vi "Labview_project.vi"() -> ()   [LabVIEW 2015]
panel:
  in  "Users":enum16{"1", "2", "3", "4"}(ring)
  out "Recived 4":bool
  out "Recived 3":bool
  out "Recived 1":bool
  out "Recived 2":bool
  out "Uncripted 4":bool
  out "Uncripted 3":bool
  out "Uncripted 2":bool
  out "Uncripted 1":bool
  out "User 4":dbl
  out "User 3":dbl
  out "User 2":dbl
  out "User 1":dbl
  in  "Hacked>Normal":bool
  in  "Data":dbl
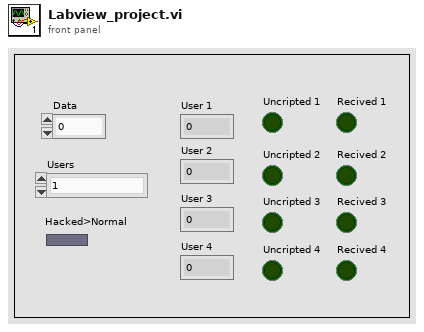
[diagram p1: front panel]
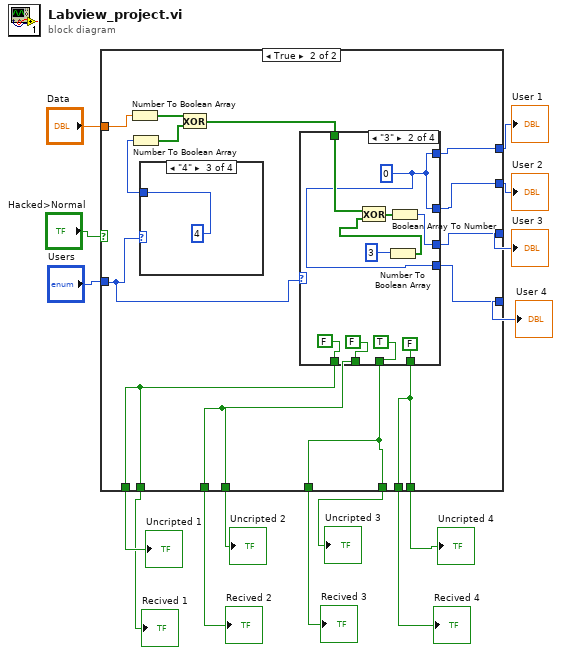
[diagram p0: block diagram]
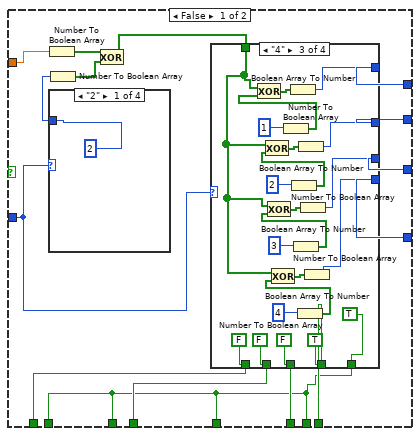
[diagram p2: hidden frame]
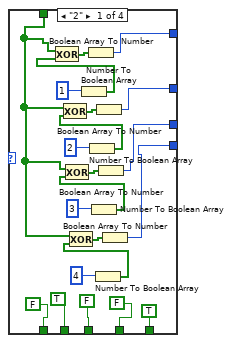
[diagram p3: hidden frame]
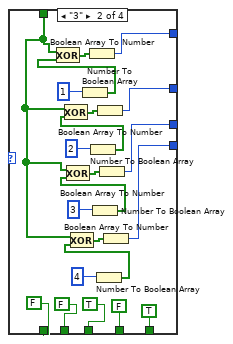
[diagram p4: hidden frame]
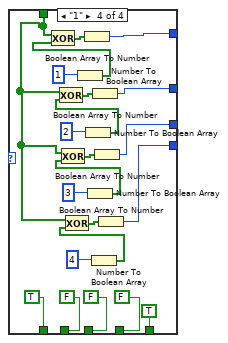
[diagram p5: hidden frame]
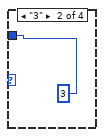
[diagram p6: hidden frame]
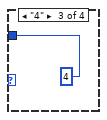
[diagram p7: hidden frame]
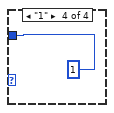
[diagram p8: hidden frame]
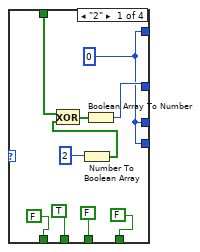
[diagram p9: hidden frame]
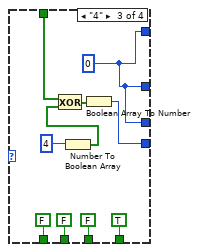
[diagram p10: hidden frame]
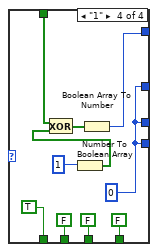
[diagram p11: hidden frame]
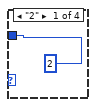
[diagram p12: hidden frame]
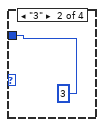
[diagram p13: hidden frame]
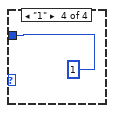
[diagram p14: hidden frame]
diagram:
  n1 = case shown="True" "Hacked>Normal" {
    tunnel: "Users" -> [w25 w132]
    tunnel: "Data" -> [w28 w134]
    tunnel: [w24 w130] -> w2
    tunnel: [w21 w129] -> w3
    tunnel: [w20 w128] -> w4
    tunnel: [w19 w127] -> w5
    tunnel: [w18 w126] -> w13
    tunnel: [w17 w125] -> w12
    tunnel: [w22 w124] -> w11
    tunnel: [w23 w123] -> w10
    tunnel: [w16 w126] -> w9
    tunnel: [w16 w125] -> w8
    tunnel: [w16 w124] -> w7
    tunnel: [w16 w123] -> w6
    frame False {
      n2 = Number To Boolean Array(number=w28) -> (Boolean array=w30:bool[])
      n3 = case shown="\"2\"" w25 {
        tunnel: [2 3 4 1] -> w27
        frame "2" {
        }
        frame "3" {
        }
        frame "4" {
        }
        frame "1" {
        }
      }
      n4 = Number To Boolean Array(number=w27) -> (Boolean array=w29:bool[])
      n5 = Exclusive Or(1:w29, 2:w30) -> (0:w26:bool[])
      n6 = case shown="\"4\"" w25 {
        tunnel: w26 -> [w36 w59 w80 w100]
        tunnel: [w32 w55 w76 w98] -> w24
        tunnel: [w33 w56 w77 w101] -> w21
        tunnel: [w34 w57 w78 w107] -> w20
        tunnel: [w35 w58 w79 w115] -> w19
        tunnel: [FALSE FALSE FALSE TRUE] -> w18
        tunnel: [TRUE FALSE FALSE FALSE] -> w17
        tunnel: [FALSE TRUE FALSE FALSE] -> w22
        tunnel: [FALSE FALSE TRUE FALSE] -> w23
        tunnel: [TRUE TRUE TRUE TRUE] -> w16
        frame "2" {
          n7 = Number To Boolean Array(number=1) -> (Boolean array=w47:bool[])
          n8 = Exclusive Or(1:w47, 2:w36) -> (0:w46:bool[])
          n9 = Boolean Array To Number(Boolean array=w46) -> (number=w35:u32)
          n10 = Number To Boolean Array(number=2) -> (Boolean array=w43:bool[])
          n11 = Exclusive Or(1:w43, 2:w36) -> (0:w44:bool[])
          n12 = Number To Boolean Array(number=3) -> (Boolean array=w38:bool[])
          n13 = Exclusive Or(1:w38, 2:w36) -> (0:w41:bool[])
          n14 = Number To Boolean Array(number=4) -> (Boolean array=w37:bool[])
          n15 = Exclusive Or(1:w37, 2:w36) -> (0:w39:bool[])
          n16 = Boolean Array To Number(Boolean array=w44) -> (number=w34:u32)
          n17 = Boolean Array To Number(Boolean array=w41) -> (number=w33:u32)
          n18 = Boolean Array To Number(Boolean array=w39) -> (number=w32:u32)
        }
        frame "3" {
          n19 = Number To Boolean Array(number=1) -> (Boolean array=w70:bool[])
          n20 = Exclusive Or(1:w70, 2:w59) -> (0:w69:bool[])
          n21 = Boolean Array To Number(Boolean array=w69) -> (number=w58:u32)
          n22 = Number To Boolean Array(number=2) -> (Boolean array=w66:bool[])
          n23 = Exclusive Or(1:w66, 2:w59) -> (0:w67:bool[])
          n24 = Number To Boolean Array(number=3) -> (Boolean array=w61:bool[])
          n25 = Exclusive Or(1:w61, 2:w59) -> (0:w64:bool[])
          n26 = Number To Boolean Array(number=4) -> (Boolean array=w60:bool[])
          n27 = Exclusive Or(1:w60, 2:w59) -> (0:w62:bool[])
          n28 = Boolean Array To Number(Boolean array=w67) -> (number=w57:u32)
          n29 = Boolean Array To Number(Boolean array=w64) -> (number=w56:u32)
          n30 = Boolean Array To Number(Boolean array=w62) -> (number=w55:u32)
        }
        frame "4" {
          n31 = Number To Boolean Array(number=1) -> (Boolean array=w91:bool[])
          n32 = Exclusive Or(1:w91, 2:w80) -> (0:w90:bool[])
          n33 = Boolean Array To Number(Boolean array=w90) -> (number=w79:u32)
          n34 = Number To Boolean Array(number=2) -> (Boolean array=w87:bool[])
          n35 = Exclusive Or(1:w87, 2:w80) -> (0:w88:bool[])
          n36 = Number To Boolean Array(number=3) -> (Boolean array=w82:bool[])
          n37 = Exclusive Or(1:w82, 2:w80) -> (0:w85:bool[])
          n38 = Number To Boolean Array(number=4) -> (Boolean array=w81:bool[])
          n39 = Exclusive Or(1:w81, 2:w80) -> (0:w83:bool[])
          n40 = Boolean Array To Number(Boolean array=w88) -> (number=w78:u32)
          n41 = Boolean Array To Number(Boolean array=w85) -> (number=w77:u32)
          n42 = Boolean Array To Number(Boolean array=w83) -> (number=w76:u32)
        }
        frame "1" {
          n43 = Number To Boolean Array(number=1) -> (Boolean array=w117:bool[])
          n44 = Exclusive Or(1:w117, 2:w100) -> (0:w116:bool[])
          n45 = Boolean Array To Number(Boolean array=w116) -> (number=w115:u32)
          n46 = Number To Boolean Array(number=2) -> (Boolean array=w108:bool[])
          n47 = Exclusive Or(1:w108, 2:w100) -> (0:w109:bool[])
          n48 = Number To Boolean Array(number=3) -> (Boolean array=w102:bool[])
          n49 = Exclusive Or(1:w102, 2:w100) -> (0:w105:bool[])
          n50 = Number To Boolean Array(number=4) -> (Boolean array=w99:bool[])
          n51 = Exclusive Or(1:w99, 2:w100) -> (0:w103:bool[])
          n52 = Boolean Array To Number(Boolean array=w109) -> (number=w107:u32)
          n53 = Boolean Array To Number(Boolean array=w105) -> (number=w101:u32)
          n54 = Boolean Array To Number(Boolean array=w103) -> (number=w98:u32)
        }
      }
    }
    frame True {
      n55 = Number To Boolean Array(number=w134) -> (Boolean array=w136:bool[])
      n56 = case shown="\"4\"" w132 {
        tunnel: [2 3 4 1] -> w133
        frame "2" {
        }
        frame "3" {
        }
        frame "4" {
        }
        frame "1" {
        }
      }
      n57 = Number To Boolean Array(number=w133) -> (Boolean array=w135:bool[])
      n58 = Exclusive Or(1:w135, 2:w136) -> (0:w131:bool[])
      n59 = case shown="\"3\"" w132 {
        tunnel: w131 -> [w144 w155 w165 w174]
        tunnel: [w137 w148 w162 w167] -> w130
        tunnel: [w137 w152 w157 w167] -> w129
        tunnel: [w142 w148 w157 w167] -> w128
        tunnel: [w137 w148 w157 w172] -> w127
        tunnel: [FALSE FALSE FALSE TRUE] -> w126
        tunnel: [TRUE FALSE FALSE FALSE] -> w125
        tunnel: [FALSE TRUE FALSE FALSE] -> w124
        tunnel: [FALSE FALSE TRUE FALSE] -> w123
        frame "2" {
          w137 = 0
          n60 = Number To Boolean Array(number=2) -> (Boolean array=w145:bool[])
          n61 = Exclusive Or(1:w145, 2:w144) -> (0:w143:bool[])
          n62 = Boolean Array To Number(Boolean array=w143) -> (number=w142:u32)
        }
        frame "3" {
          w148 = 0
          n63 = Number To Boolean Array(number=3) -> (Boolean array=w154:bool[])
          n64 = Exclusive Or(1:w154, 2:w155) -> (0:w153:bool[])
          n65 = Boolean Array To Number(Boolean array=w153) -> (number=w152:u32)
        }
        frame "4" {
          w157 = 0
          n66 = Number To Boolean Array(number=4) -> (Boolean array=w164:bool[])
          n67 = Exclusive Or(1:w164, 2:w165) -> (0:w163:bool[])
          n68 = Boolean Array To Number(Boolean array=w163) -> (number=w162:u32)
        }
        frame "1" {
          w167 = 0
          n69 = Number To Boolean Array(number=1) -> (Boolean array=w175:bool[])
          n70 = Exclusive Or(1:w175, 2:w174) -> (0:w173:bool[])
          n71 = Boolean Array To Number(Boolean array=w173) -> (number=w172:u32)
        }
      }
    }
  }
  "User 1" <- w5
  "User 2" <- w4
  "User 3" <- w3
  "User 4" <- w2
  "Uncripted 2" <- w12
  "Uncripted 1" <- w13
  "Uncripted 3" <- w11
  "Uncripted 4" <- w10
  "Recived 2" <- w8
  "Recived 1" <- w9
  "Recived 3" <- w7
  "Recived 4" <- w6
